vi "ParseAuthority.vi"(11 "authority":string) -> (0 "password":string, 1 "username":string, 2 "port":string, 3 "host":string)   [LabVIEW 2013, in "openURI.lvlib"]
uses:
  openURI.lvlib
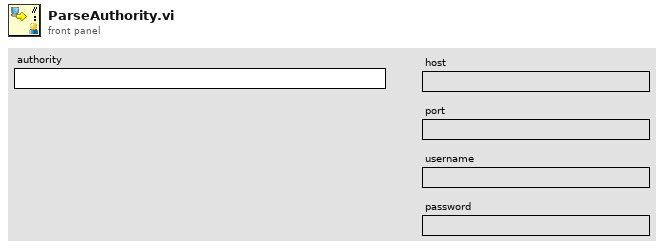
[diagram p1: front panel]
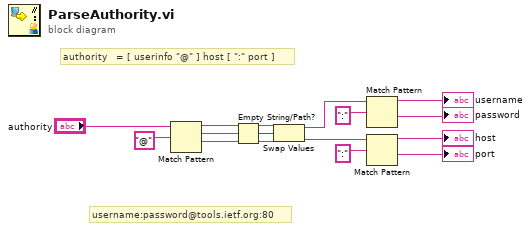
[diagram p0: block diagram]
diagram:
  # "username:password@tools.ietf.org:80"
  # "authority   = [ userinfo \"@\" ] host [ \":\" port ]"
  n1 = Match Pattern(string="authority", regular expression="@") -> (before substring=w10:string, match substring=w12:string, after substring=w9:string)  [unwired: 1 in, 1 out]
  n2 = Empty String/Path?(string/path=w12) -> (empty?=w11:bool)
  n3 = Swap Values(12:w10, 13:w11, 14:w9) -> (1:w7:string, 3:w4:string)
  n4 = Match Pattern(string=w7, regular expression=":") -> (before substring=→"username":string, after substring=→"password":string)  [unwired: 1 in, 2 out]
  n5 = Match Pattern(string=w4, regular expression=":") -> (before substring=→"host":string, after substring=→"port":string)  [unwired: 1 in, 2 out]
